vi "GetFirstScreen.vi"(8 "error in (no error)":errorcluster, 11 "Game in":refnum<class "Game.lvclass">) -> (0 "error out":errorcluster, 2 "Array":u32[][](array[numeric]), 3 "Game out":refnum<class "Game.lvclass">)   [LabVIEW 2019, in "RT_Game.lvlib" / "Game.lvclass"]
uses:
  Game.lvclass
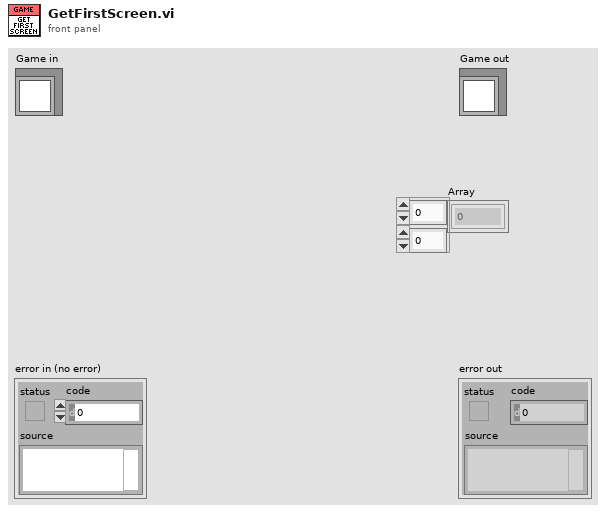
[diagram p1: front panel]
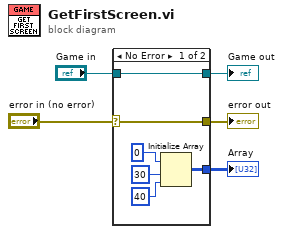
[diagram p0: block diagram]
diagram:
  n1 = case shown="No Error" "error in (no error)" {
    selector: "error in (no error)" -> [w10 w13]
    tunnel: [w10 w13] -> w4
    tunnel: [w11 w12] -> w2
    tunnel: "Game in" -> [w11 w12]
    tunnel: [w6 _] -> w1
    frame No Error {
      n2 = Initialize Array(0 ("Numeric"), 30 ("dimension size"), 40 ("dimension size")) -> (w6:i32[][])
    }
    frame Error {
    }
  }
  "error out" <- w4
  "Game out" <- w2
  "Array" <- w1
